vi "test_Set-Get Protocol VISA.vi"(8 "error in (no error)":errorcluster, 11 "TestCase in":refnum<class "Instrument Addon Scripting API Custom Device Unit Tests.lvclass">) -> (0 "error out":errorcluster, 3 "TestCase out":refnum<class "Instrument Addon Scripting API Custom Device Unit Tests.lvclass">)   [LabVIEW 2019, in "Instrument Addon Scripting API Custom Device Unit Tests.lvclass"]
uses:
  Instrument Addon Scripting API Custom Device Unit Tests.lvclass
  Includes/Protocols.lvlibp/VISA/VISA.lvclass
  C:/Users/nitest/Desktop/Git/niveristand-instrument-addon-custom-device/Includes/Protocols.lvlibp/Protocol Parent/Protocol Parent.lvclass
  Includes/Protocols.lvlibp/AK RS-xxx/AK RS-xxx.lvclass
  Instrument Addon Scripting API Custom Device Unit Tests.lvclass/Instrument Addon Scripting API Custom Device Unit Tests.ctl
  Includes/Protocols.lvlibp/VISA/Data Access/Write Append Write Termination Character.vi
  Includes/Protocols.lvlibp/VISA/Data Access/Write Enable Termination Character.vi
  Includes/Protocols.lvlibp/VISA/Data Access/Write Termination Character.vi
  Includes/Protocols.lvlibp/VISA/Data Access/Write Timeout.vi
  Includes/Protocols.lvlibp/VISA/Data Access/Write VISA Resource.vi
  Instrument Addon Scripting API Test Assets/Instrument Addon Scripting API Test Assets.lvclass
  <vilib>/addons/_JKI Toolkits/VI Tester/TestCase.llb/TestCase.lvclass
  APIs/Scripting API/Instrument Addon Scripting API.lvlib
  C:/Program Files (x86)/National Instruments/LabVIEW 2019/vi.lib/addons/_JKI Toolkits/VI Tester/TestCase.llb/TestCase.lvclass
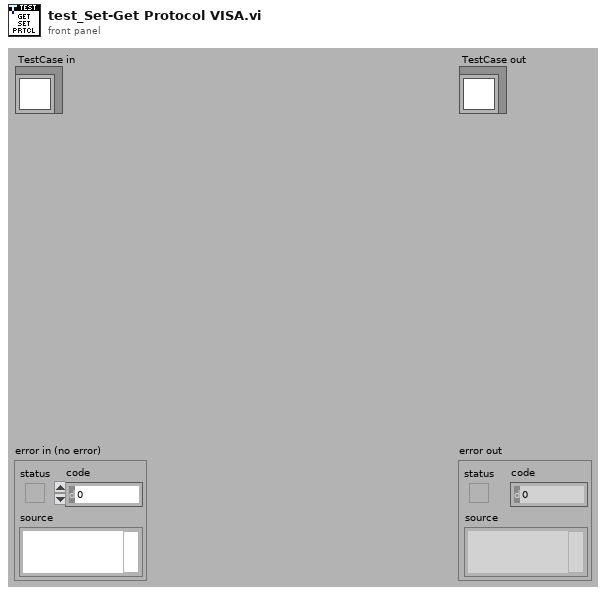
[diagram p1: front panel]
types:
  T1 = typedef "Custom Device API.lvlib/Custom Device Item Ref.ctl" = u64
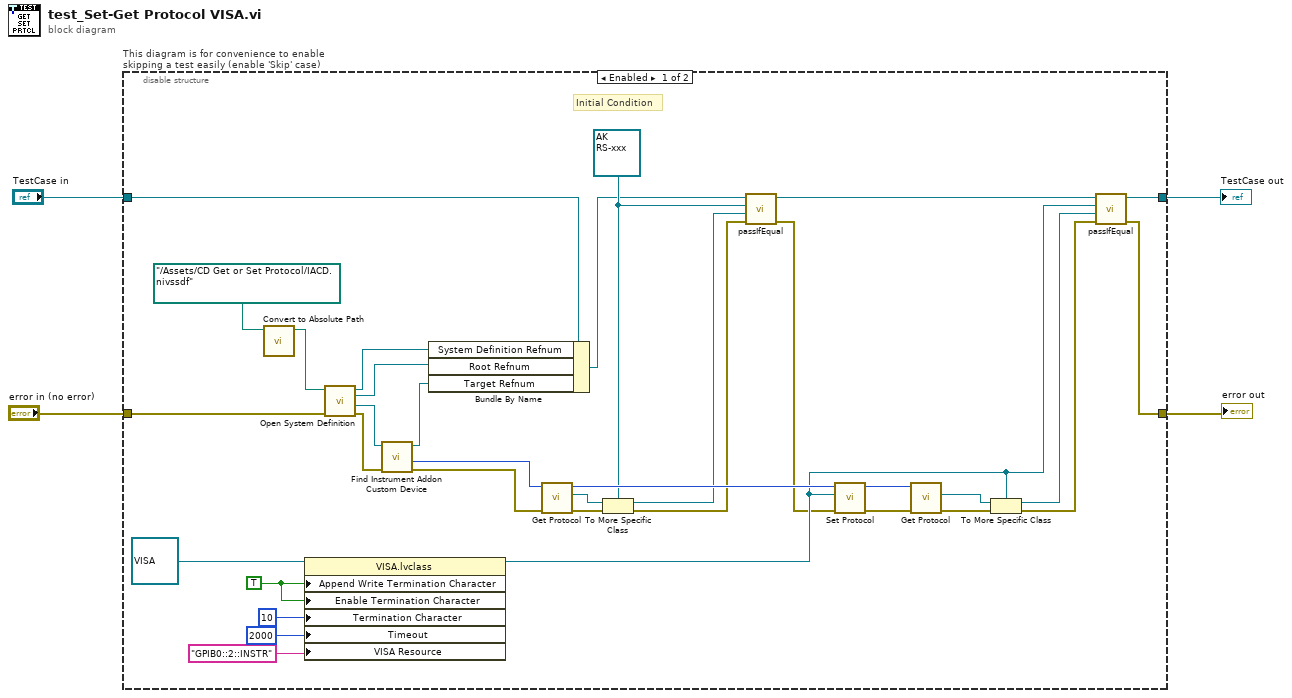
[diagram p0: block diagram]
diagram:
  n1 = disable-structure "This diagram is for convenience to enable skipping a test easily (enable 'Skip' case)" shown="Enabled" {
    disable-tunnel: "TestCase in" -> [w9 w42]
    disable-tunnel: [w27 w40] -> w1
    disable-tunnel: [w25 w41] -> w3
    disable-tunnel: "error in (no error)" -> [w38 w39]
    frame Enabled {
      w11 = refnum<class "AK RS-xxx.lvclass"> refnum ("reference out")
      w32 = TRUE
      # "Initial Condition"
      n2 = call "Convert to Absolute Path.vi"("System Definition File"=path "../Assets/CD Get or Set Protocol/IACD.nivssdf" ("SDF file")) -> ("Absolute Path"=w36:path)  [unwired: 10 in]
      n3 = property class="VISA.lvclass"(reference=refnum<class "VISA.lvclass"> refnum ("Protocols.lvlibp:VISA.lvclass"), "Append Write Termination Character"=w32, "Enable Termination Character"=w32, "Termination Character"=u8 10, "Timeout"=u32 2000, "VISA Resource"="GPIB0::2::INSTR") -> (reference out=w17:refnum<class "VISA.lvclass">)  [unwired: 1 in, 1 out]
      n4 = call "Open System Definition.vi"("error in (no error)"=w38, "System Definition File"=w36) -> ("error out"=w35:errorcluster, "Target Refnum"=w34:refnum<k24>, "Root Refnum"=w6:refnum<k24>, "System Definition Refnum"=w7:refnum<k24>)  [unwired: 6 in]
      n5 = call "Find Instrument Addon Custom Device.vi"("error in"=w35, "target in"=w34) -> ("error out"=w24:errorcluster, "NodeID"=w23:u64, "target out"=w5:refnum<k24>)  [unwired: 7 in]
      n6 = Bundle By Name(cluster=w9, "System Definition Refnum"=w7, "Root Refnum"=w6, "Target Refnum"=w5) -> (w8:refnum<class "Instrument Addon Scripting API Custom Device Unit Tests.lvclass">)
      n7 = call "Get Protocol.vi"("error in (no error)"=w24, "instrument addon refnum in"=w23) -> ("error out"=w14:errorcluster, "protocol"=w13:refnum<class "Protocol Parent.lvclass">, "instrument addon refnum out"=w18:T1)  [unwired: 7 in]
      n8 = To More Specific Class(target class=w11, reference=w13, error in=w14) -> (specific class reference=w12:refnum<class "AK RS-xxx.lvclass">, error out=w10:errorcluster)
      n9 = call-dynamic "passIfEqual.vi"("error in (no error)"=w10, "y"=w12, "x"=w11, "TestCase in"=w8) -> ("error out"=w15:errorcluster, "TestCase out"=w16:refnum<class "Instrument Addon Scripting API Custom Device Unit Tests.lvclass">)  [unwired: 6 in]
      n10 = call "Set Protocol.vi"("error in (no error)"=w15, "protocol"=w17, "instrument addon refnum in"=w18) -> ("error out"=w21:errorcluster, "instrument addon refnum out"=w22:T1)  [unwired: 7 in]
      n11 = call "Get Protocol.vi"("error in (no error)"=w21, "instrument addon refnum in"=w22) -> ("error out"=w19:errorcluster, "protocol"=w20:refnum<class "Protocol Parent.lvclass">)  [unwired: 7 in, 1 out]
      n12 = To More Specific Class(target class=w17, reference=w20, error in=w19) -> (specific class reference=w26:refnum<class "VISA.lvclass">, error out=w28:errorcluster)
      n13 = call-dynamic "passIfEqual.vi"("error in (no error)"=w28, "y"=w26, "x"=w17, "TestCase in"=w16) -> ("error out"=w25:errorcluster, "TestCase out"=w27:refnum<class "Instrument Addon Scripting API Custom Device Unit Tests.lvclass">)  [unwired: 6 in]
    }
    frame Disabled {
      # "skip test result while test is under development"
      n14 = call <vilib>:"skip.vi"("error in (no error)"=w39, "TestCase in"=w42) -> ("error out"=w41:errorcluster, "TestCase out"=w40:refnum<class "Instrument Addon Scripting API Custom Device Unit Tests.lvclass">)  [unwired: 8 in]
    }
  }
  "error out" <- w3
  "TestCase out" <- w1
